vi "generate_timestamp.vi"(0 "data in":dbl[][](array[numeric]), 1 "Set threshold on standard deviation":bool, 5 "interval time (s)":dbl, 7 "time stamp in":timestamp format="%<%I:%M %p %d/%m/%Y>T", 9 "index in":i32, 11 "Sampling rate (Hz)":dbl=5000.0, 12 "Threshold of standard deviation":dbl) -> (2 "mean values":dbl[](array[numeric]), 3 "standard deviation":dbl[](array[numeric]), 4 "data out":dbl[][](array[numeric]), 6 "time stamp out":timestamp format="%<%I:%M %p %d/%m/%Y>T", 8 "data averaged":bool, 10 "index out":i32, 13 "min values":dbl[](array[numeric]), 14 "max values":dbl[](array[numeric]), 15 "data with time":dbl[][](array[numeric]))   [LabVIEW 2018]
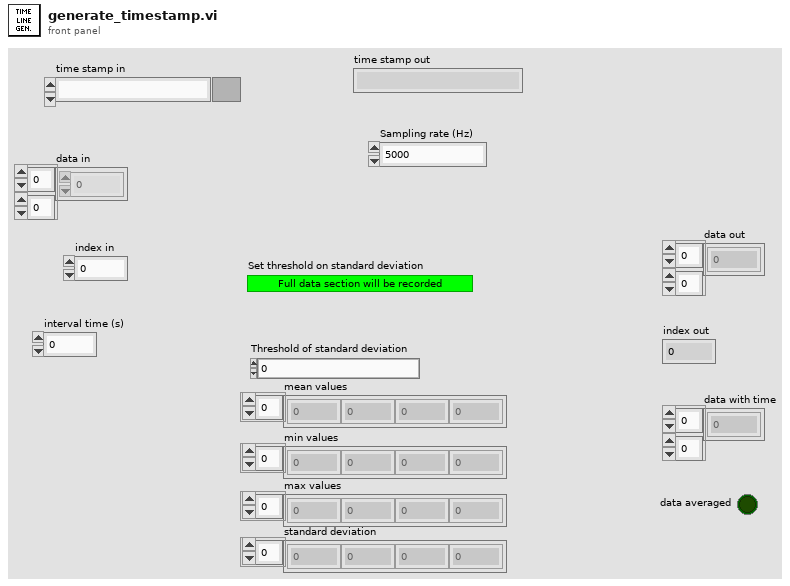
[diagram p1: front panel]
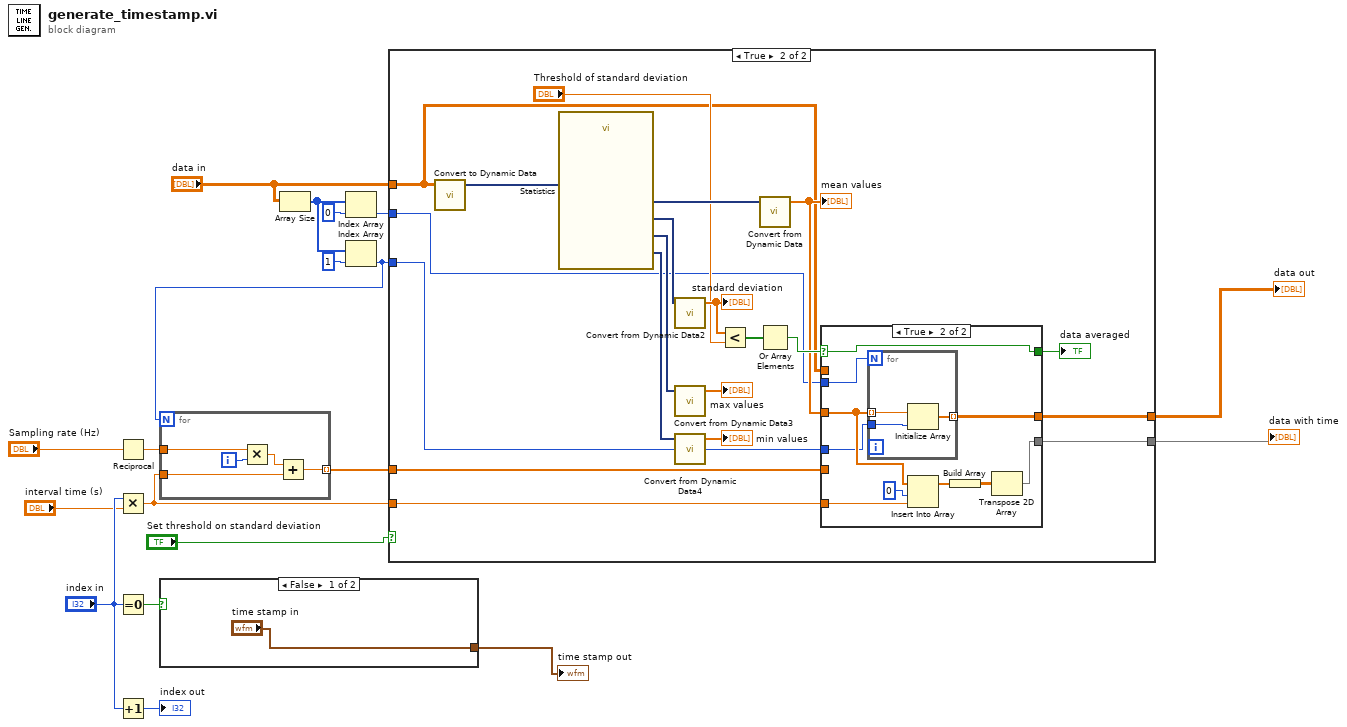
[diagram p0: block diagram]
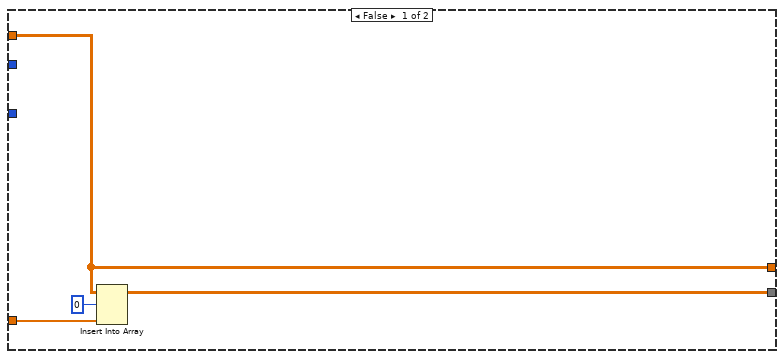
[diagram p2: hidden frame]
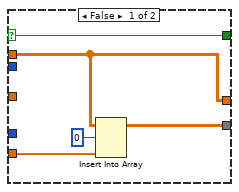
[diagram p3: hidden frame]
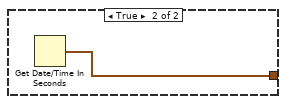
[diagram p4: hidden frame]
diagram:
  n1 = Reciprocal(x="Sampling rate (Hz)") -> (1/x=w15:dbl)
  n2 = Multiply(x="index in", y="interval time (s)") -> (x*y=w16:dbl)
  n3 = Equal To 0?(x="index in") -> (x = 0?=w18:bool)
  n4 = Increment(x="index in") -> (x+1=→"index out":i32)
  n5 = case shown="False" w18 {
    tunnel: ["time stamp in" w20] -> w1
    frame False {
    }
    frame True {
      n6 = Get Date/Time In Seconds() -> (seconds since 1Jan1904=w20:timestamp)
    }
  }
  "time stamp out" <- w1
  n7 = Array Size(array="data in") -> (size(s)=w11:i32[])
  n8 = Index Array(array=w11, index=0) -> (element=w10:i32)
  n9 = Index Array(array=w11, index=1) -> (element=w2:i32)
  n10 = for {
    N: w2 -> [_]
    tunnel: w16 -> [w22]
    tunnel: w15 -> [w25]
    tunnel: [w21] -> w17 mode=indexing
    i -> [w24]
    n11 = Multiply(x=w25, y=w24) -> (x*y=w23:dbl)
    n12 = Add(x=w23, y=w22) -> (x+y=w21:dbl)
  }
  n13 = case shown="True" "Set threshold on standard deviation" {
    tunnel: [w26 w37] -> w3
    tunnel: w16 -> [_ w36]
    tunnel: w17 -> [w29 w35]
    tunnel: [w27 w34] -> w4
    tunnel: "data in" -> [w27 w32]
    tunnel: w2 -> [_ w31]
    tunnel: w10 -> [_ w30]
    frame False {
      n14 = Insert Into Array(array=w27, index (row)=0, new element=w29) -> (w26:dbl[][])  [unwired: 1 in]
    }
    frame True {
      n15 = call "Convert to Dynamic Data"("2D Array"=w32) -> ("Dynamic Data Type"=w48:dynamicdata)  [unwired: 3 in]
      n16 = call "Statistics"("Signals"=w48) -> ("Standard Dev"=w47:dynamicdata, "Arithmetic Mean"=w49:dynamicdata, "Minimum"=w45:dynamicdata, "Maximum"=w46:dynamicdata)  [unwired: 22 in, 1 out]
      n17 = call "Convert from Dynamic Data2"("Dynamic Data Type"=w47) -> ("Array"=w42:dbl[])  [unwired: 3 in]
      "standard deviation" <- w42
      n18 = call "Convert from Dynamic Data3"("Dynamic Data Type"=w46) -> ("Array"=→"max values":dbl[])  [unwired: 3 in]
      n19 = call "Convert from Dynamic Data4"("Dynamic Data Type"=w45) -> ("Array"=→"min values":dbl[])  [unwired: 3 in]
      n20 = Less?(x=w42, y="Threshold of standard deviation") -> (x < y?=w40:bool[])
      n21 = call "Convert from Dynamic Data"("Dynamic Data Type"=w49) -> ("Array"=w38:dbl[])  [unwired: 3 in]
      "mean values" <- w38
      n22 = Or Array Elements(Boolean array=w40) -> (logical OR=w39:bool)
      n23 = case shown="True" w39 {
        selector: w39 -> [w52 w61]
        tunnel: w38 -> [_ w64]
        tunnel: [w51 w58] -> w37
        tunnel: w36 -> [_ w62]
        tunnel: w35 -> [w53 _]
        tunnel: [w50 w57] -> w34
        tunnel: [w52 w61] -> w33
        tunnel: w32 -> [w50 _]
        tunnel: w31 -> [_ w56]
        tunnel: w30 -> [_ w55]
        frame False {
          n24 = Insert Into Array(array=w50, index (row)=0, new element=w53) -> (w51:dbl[][])  [unwired: 1 in]
        }
        frame True {
          n25 = for {
            N: w55 -> [_]
            tunnel: w64 -> [w67] mode=indexing
            tunnel: [w66] -> w57 mode=indexing
            tunnel: w56 -> [w65]
            n26 = Initialize Array(w67, w65) -> (w66:dbl[])
          }
          n27 = Insert Into Array(array=w64, index=0, new element=w62) -> (w60:dbl[])
          n28 = Build Array(w60) -> (w59:dbl[][])
          n29 = Transpose 2D Array(2D array=w59) -> (transposed array=w58:dbl[][])
        }
      }
      "data averaged" <- w33
    }
  }
  "data with time" <- w3
  "data out" <- w4
